vi "logic settings buffer.vi"(0 "output settings":T5, 1 "Rules":T6=[{"state rules"=[{"next state"=0, "conditions"=[], "number of conditions"=1, "Rule name"="New rule"}], "State name"="New state"}] {"state rules"."number of conditions" min=1 step=1; "state rules"."conditions"."Data average interval" min=0.0 format="%^#_3g"; "state rules"."conditions"."sensors and variables" items=["Elapsed time in current state"]; "state rules"."next state" items=["down flow", "Backwash", ""]}, 3 "output descriptions":string[][](array[string]), 4 "index":i32, 5 "Plant  state":i16(ring), 6 "Elapsed time in current state":dbl format="%.2f", 7 "command":T11=enum."write all", 8 "Set Points":T2[](array[typedef])=[{"name"="", "unit"="", "value"=0.0, "Type"=enum."Constant", "variable"={"selected sensors"=[], "selected set points"=[], "VI"=path "", "Data average interval"=0.0, "code ref"=refnum}}] {"value" format="%#_6p"; "variable"."Data average interval" min=0.0 format="%^#_3g"}, 11 "rule file in":path) -> (10 "Setpoint match":T1[](array[typedef]), 12 "Set Points out":T2[](array[typedef])=[{"name"="", "unit"="", "value"=0.0, "Type"=enum."Constant", "variable"={"selected sensors"=[], "selected set points"=[], "VI"=path "", "Data average interval"=0.0, "code ref"=refnum}}] {"value" format="%#_6p"; "variable"."Data average interval" min=0.0 format="%^#_3g"}, 13 "rule file out":path, 14 "ouput settings out":T5, 15 "Rules out":T6=[{"state rules"=[{"next state"=0, "conditions"=[], "number of conditions"=1, "Rule name"="New rule"}], "State name"="New state"}] {"state rules"."number of conditions" min=1 step=1; "state rules"."conditions"."Data average interval" min=0.0 format="%^#_3g"; "state rules"."conditions"."sensors and variables" items=["Elapsed time in current state"]; "state rules"."next state" items=["down flow", "Backwash", ""]}, 17 "output descriptions out":string[][](array[string]), 18 "code error array":errorcluster[](array[cluster]), 19 "Plant  state out":u16(ring)=1)   [LabVIEW 2012]
uses:
  logic buffer cmd.ctl
  rules.ctl
  State rules.ctl
  rule.ctl
  condition.ctl
  greater or less.ctl
  Output control.ctl
  variable setpoint.ctl
  data ave interval.ctl
  type specifier for control code.ctl
  setpoint match.ctl
  DAQ configuration/Sensor buffer command.ctl
  file/file action.ctl
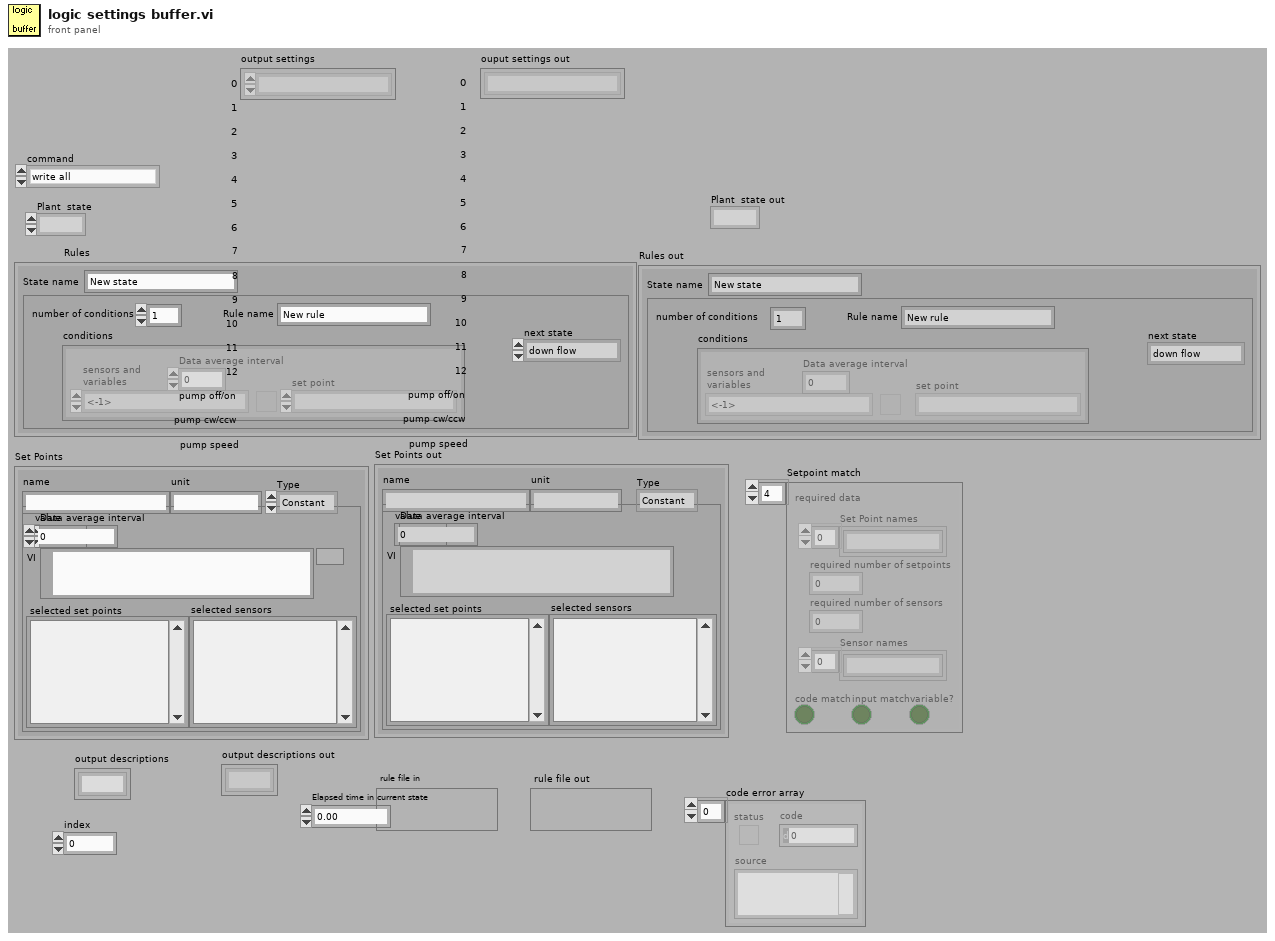
[diagram p1: front panel]
types:
  T1 = typedef "setpoint match.ctl" = cluster{"required data":cluster{"Set Point names":string[], "required number of setpoints":u8, "required number of sensors":u8, "Sensor names":string[]}, "input match":bool, "code match":bool, "variable?":bool}
  T2 = typedef "variable setpoint.ctl" = cluster{"name":string, "unit":string, "value":dbl, "Type":enum16{"Constant", "Variable"}, "variable":cluster{"selected sensors":i32[], "selected set points":i32[], "VI":path, "Data average interval":T3, "code ref":T4}}
  T3 = typedef "data ave interval.ctl" = dbl
  T4 = typedef "type specifier for control code.ctl" = refnum<vi>
  T5 = typedef "Output control.ctl" = u16[][]
  T6 = typedef "rules.ctl" = T7[]
  T7 = typedef "State rules.ctl" = cluster{"state rules":T8[], "State name":string}
  T8 = typedef "rule.ctl" = cluster{"next state":u16, "conditions":T9[], "number of conditions":u8, "Rule name":string}
  T9 = typedef "condition.ctl" = cluster{"> or <":T10, "set point":i32, "sensors and variables":i32, "Data average interval":dbl}
  T10 = typedef "greater or less.ctl" = bool
  T11 = typedef "logic buffer cmd.ctl" = enum16{"read", "write ouput settings", "write rules", "write setpoints", "write output descriptions", "write all", "calculate setpoints", "save", "open", "Load all setpoint code", "Load one setpoint code", "Configure one setpoint code"}
  T12 = typedef "Sensor buffer command.ctl" = enum16{"read average", "read recent", "read all", "write", "configure", "clear"}
  T13 = typedef "file action.ctl" = enum16{"Save", "Open"}
  T14 = typedef "Sensor data.ctl" = cluster{" Sensor array":T15[], "Time":dbl}
  T15 = typedef "sensor cluster.ctl" = cluster{"voltage":sgl, "scaled":sgl, "units":string, "Out of Range":bool}
  T16 = cluster{"Set Points out":T2[], "Rules":T6, "s? t:f":T5, "output descriptions":string[][]}
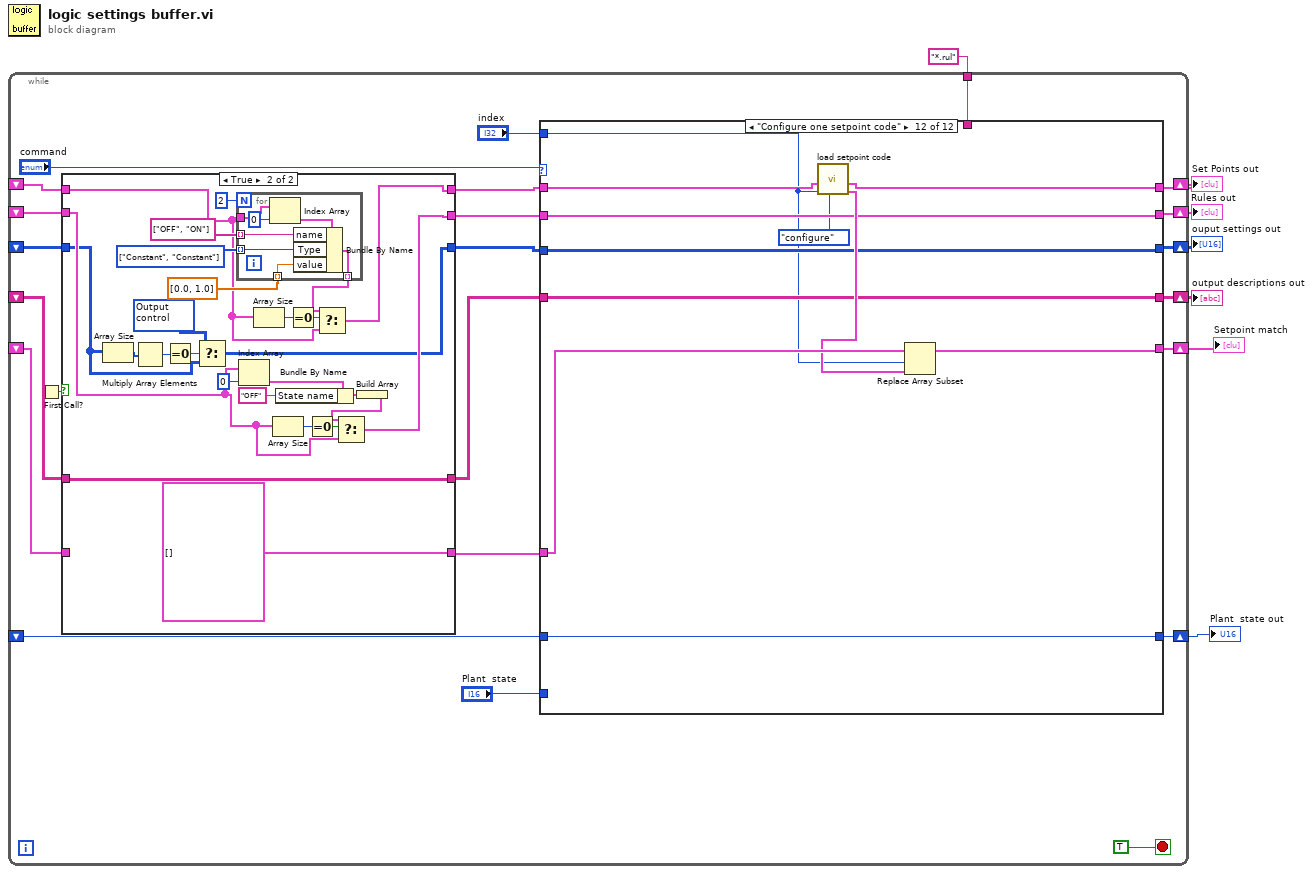
[diagram p0: block diagram]
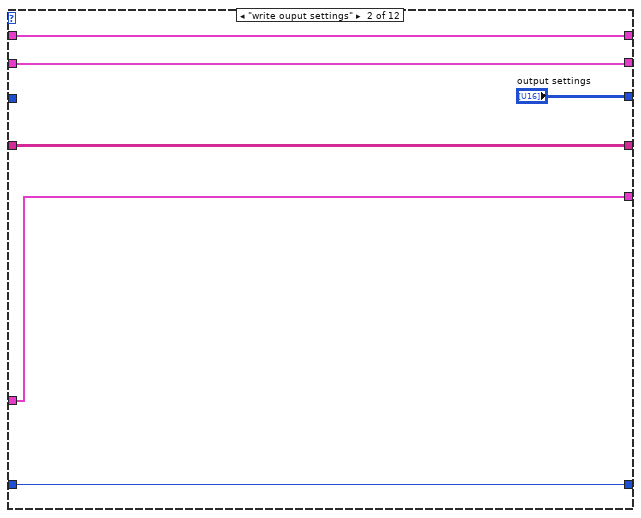
[diagram p4: hidden frame]
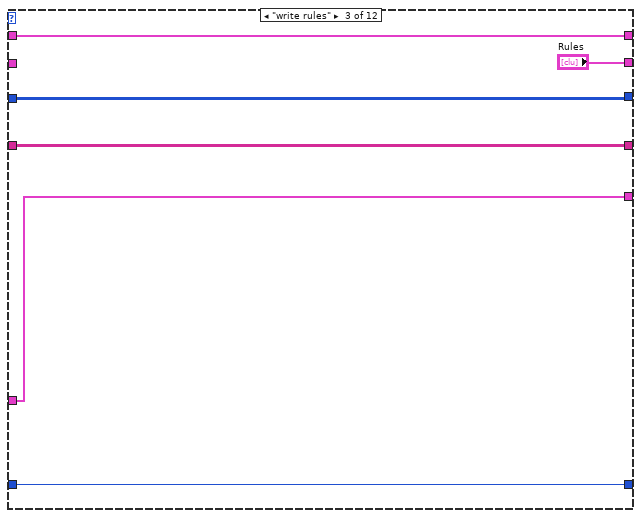
[diagram p5: hidden frame]
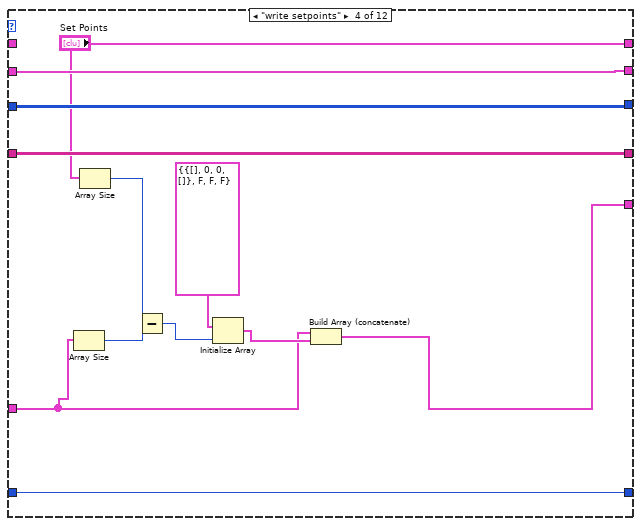
[diagram p6: hidden frame]
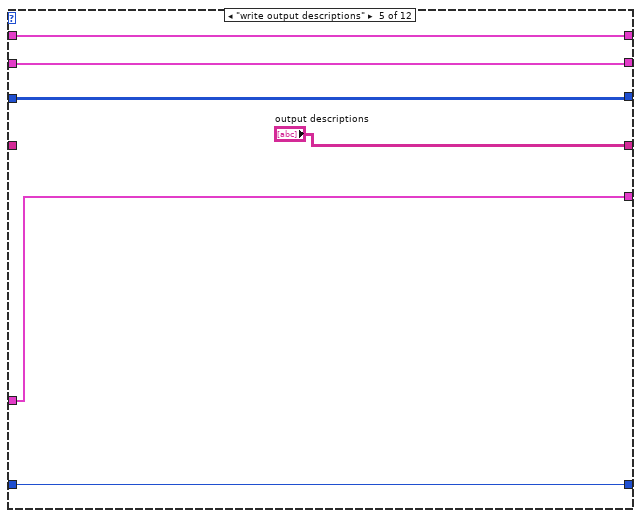
[diagram p7: hidden frame]
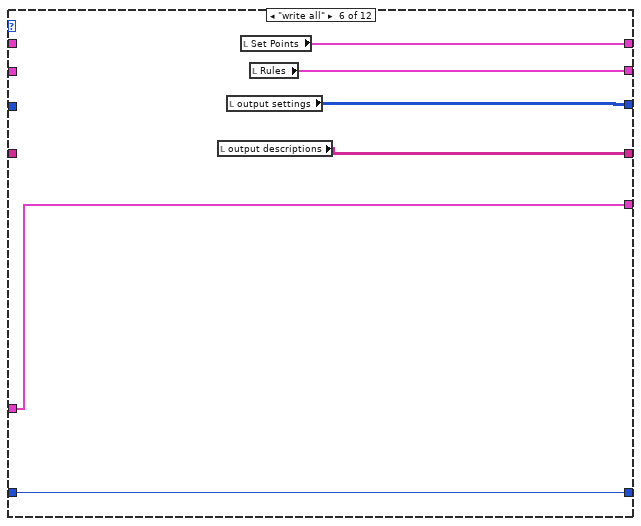
[diagram p8: hidden frame]
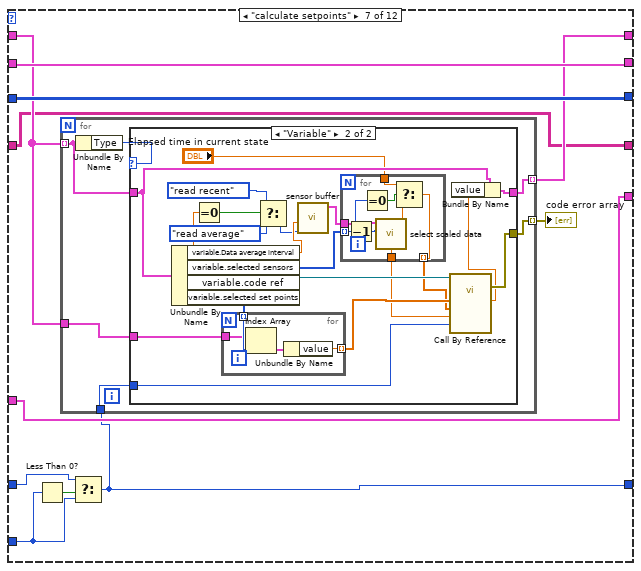
[diagram p9: hidden frame]
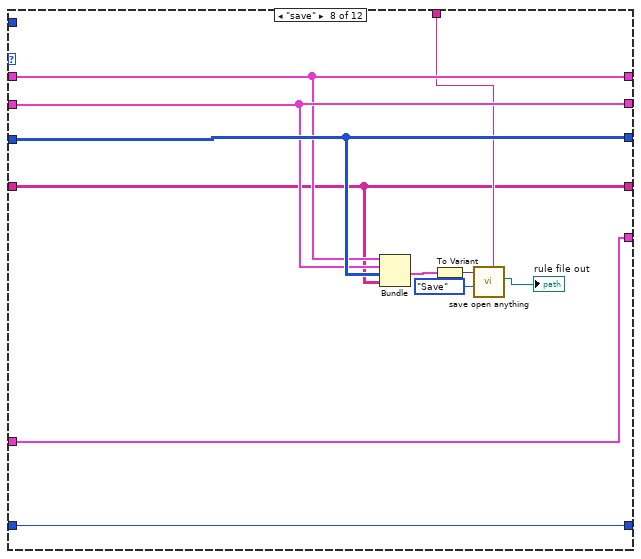
[diagram p11: hidden frame]
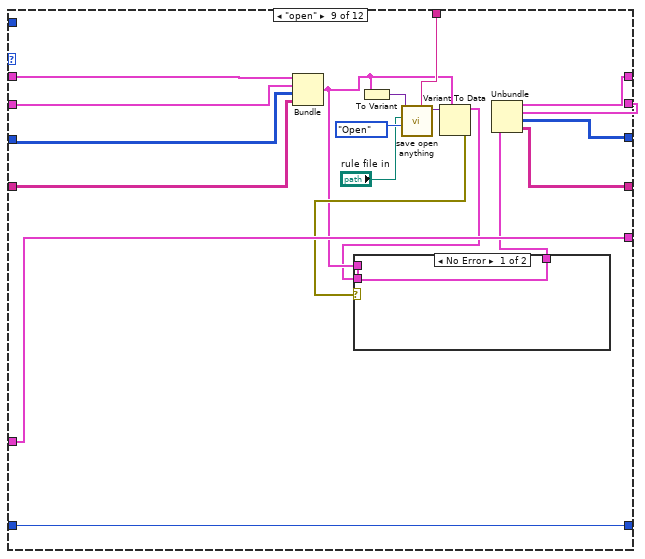
[diagram p12: hidden frame]
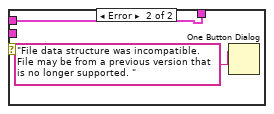
[diagram p13: hidden frame]
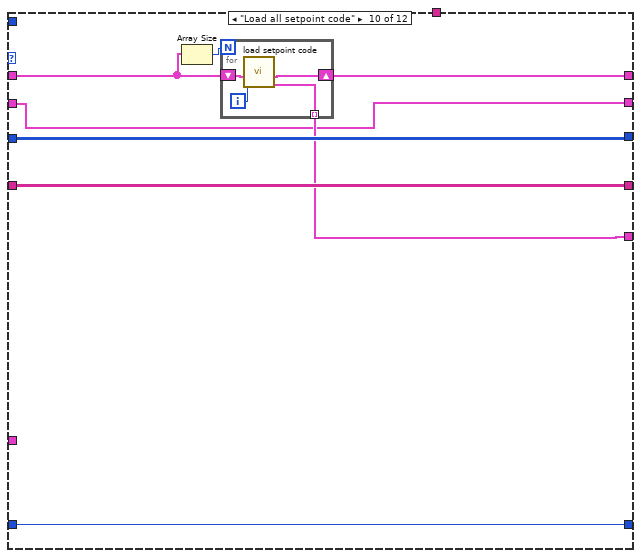
[diagram p14: hidden frame]
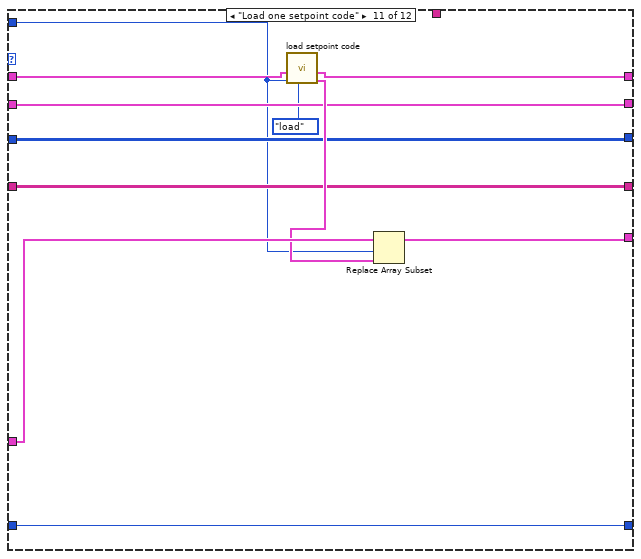
[diagram p15: hidden frame]
diagram:
  n1 = while {
    shift-right: [w29] -> w6
    shift-left: _ -> [w21]
    shift-right: [w30] -> w7
    shift-left: _ -> [w23]
    shift-right: [w15] -> w5
    shift-left: _ -> [w19]
    tunnel: "*.rul" ("pattern") -> [w27]
    shift-right: [w18] -> w3
    shift-left: _ -> [w17]
    shift-right: [w14] -> w2
    shift-left: _ -> [w12]
    shift-right: [w10] -> w1
    shift-left: _ -> [w11]
    stop <- TRUE stop-if-true
    n2 = First Call?() -> (First Call?: T/F=w25:bool)
    n3 = case shown="True" w25 {
      tunnel: [w35 w39] -> w24
      tunnel: w23 -> [w35 w38]
      tunnel: [w34 w40] -> w22
      tunnel: w21 -> [w34 w41]
      tunnel: [w33 w42] -> w20
      tunnel: w19 -> [w33 w43]
      tunnel: [w32 w37] -> w16
      tunnel: w17 -> [w32 w37]
      tunnel: [w31 T1[] [] ("Setpoint match")] -> w13
      tunnel: w12 -> [w31 _]
      frame False {
      }
      frame True {
        w52 = enum16{"Constant", "Variable"}[] [enum."Constant", enum."Constant"] items=["Constant", "Variable"]
        w58 = T5 [[0], [0], [0], [0], [0], [0], [0], [0], [0], [0], [0], [0], [0], [0], [0], [0], [0], [0], [0], [0], [0], [0], [0], [0], [0], [0], [0], [0], [0], [0], [0], [0]] items=[""] ("s? t:f")
        n4 = Array Size(array=w38) -> (size(s)=w61:i32[])
        n5 = Multiply Array Elements(1:w61) -> (0:w60:i32)
        n6 = Equal To 0?(x=w60) -> (x = 0?=w59:bool)
        n7 = Select(t=w58, s=w59, f=w38) -> (s? t:f=w39:T5)
        n8 = for {
          N: 2 -> [_]
          tunnel: w43 -> [w64]
          tunnel: [w68] -> w54 mode=indexing
          tunnel: string[] ["OFF", "ON"] -> [w67] mode=indexing
          tunnel: w52 -> [w66] mode=indexing
          tunnel: dbl[] [0.0, 1.0] -> [w65] mode=indexing
          n9 = Index Array(array=w64, index=0) -> (element=w62:T2)
          n10 = Bundle By Name(cluster=w62, "name"=w67, "Type"=w66, "value"=w65) -> (w68:T2)
        }
        n11 = Index Array(array=w41, index=0) -> (element=w47:T7)
        n12 = Array Size(array=w43) -> (size(s)=w56:i32)
        n13 = Array Size(array=w41) -> (size(s)=w50:i32)
        n14 = Bundle By Name(cluster=w47, "State name"="OFF") -> (w46:T7)
        n15 = Equal To 0?(x=w56) -> (x = 0?=w57:bool)
        n16 = Equal To 0?(x=w50) -> (x = 0?=w49:bool)
        n17 = Select(t=w54, s=w57, f=w43) -> (s? t:f=w42:T2[])
        n18 = Build Array(w46) -> (w45:T7[])
        n19 = Select(t=w45, s=w49, f=w41) -> (s? t:f=w40:T6)
      }
    }
    n20 = case shown="\"Configure one setpoint code\"" "command" {
      tunnel: [w73 "output settings" w85 w97 w102 w108 w121 w168 w180 w197 w209 w220] -> w30
      tunnel: [w74 w80 "Rules" w98 w103 w109 w120 w167 w184 w194 w210 w221] -> w29
      tunnel: w22 -> [w74 w80 _ w98 w103 _ w120 w167 w187 w194 w210 w221]
      tunnel: w24 -> [w73 _ w85 w97 w102 _ w121 w168 w186 w197 w209 w220]
      tunnel: [w72 w79 w84 "Set Points" w104 w110 w119 w166 w179 w198 w214 w225] -> w15
      tunnel: w20 -> [w72 w79 w84 _ w104 _ w118 w166 w185 w199 w215 w226]
      tunnel: w27 -> [_ _ _ _ _ _ _ w165 w182 _ _ _]
      tunnel: [w71 w77 w83 w96 "output descriptions" w107 w116 w162 w177 w196 w208 w219] -> w18
      tunnel: w16 -> [w71 w77 w83 w96 _ _ w116 w162 w178 w196 w208 w219]
      tunnel: [w70 w76 w82 w88 w100 w106 w115 w161 w176 w195 w212 w223] -> w14
      tunnel: w13 -> [w70 w76 w82 w89 w100 w106 w115 w161 w176 _ w213 w224]
      tunnel: w11 -> [w69 w75 w81 w87 w99 w105 w112 w160 w171 w193 w207 w218]
      tunnel: [w69 w75 w81 w87 w99 w105 w113 w160 w171 w193 w207 w218] -> w10
      tunnel: "Plant  state" -> [_ _ _ _ _ _ w111 _ _ _ _ _]
      tunnel: "index" -> [_ _ _ _ _ _ _ _ _ _ w205 w216]
      frame "read", Default {
      }
      frame "write ouput settings" {
      }
      frame "write rules" {
      }
      frame "write setpoints" {
        n21 = Array Size(array=w89) -> (size(s)=w92:i32)
        n22 = Array Size(array="Set Points") -> (size(s)=w94:i32)
        n23 = Subtract(x=w94, y=w92) -> (x-y=w93:i32)
        n24 = Initialize Array(T1 {"required data"={"Set Point names"=[], "required number of setpoints"=0, "required number of sensors"=0, "Sensor names"=[]}, "input match"=FALSE, "code match"=FALSE, "variable?"=FALSE} ("setpoint match"), w93) -> (w90:T1[])
        n25 = Build Array (concatenate)(w89, w90) -> (w88:T1[])
      }
      frame "write output descriptions" {
      }
      frame "write all" {
        n26 = local read "output descriptions"() -> (w107:string[][])
        n27 = local read "output settings"() -> (w108:T5)
        n28 = local read "Set Points"() -> (w110:T2[])
        n29 = local read "Rules"() -> (w109:T6)
      }
      frame "calculate setpoints" {
        n30 = Less Than 0?(x=w111) -> (x < 0?=w114:bool)
        n31 = Select(t=w112, s=w114, f=w111) -> (s? t:f=w113:i16)
        n32 = for {
          tunnel: [w127] -> w117 mode=indexing
          tunnel: w118 -> [w125] mode=indexing
          tunnel: [w124] -> w119 mode=indexing
          tunnel: w118 -> [w123]
          tunnel: w113 -> [w122]
          n33 = Unbundle By Name(w125) -> ("Type"=w126:enum16{"Constant", "Variable"})
          n34 = case shown="\"Variable\"" w126 {
            tunnel: [_ w147] -> w127
            tunnel: w122 -> [_ w146]
            tunnel: w125 -> [w128 w132]
            tunnel: [w128 w133] -> w124
            tunnel: w123 -> [_ w134]
            frame "Constant", Default {
            }
            frame "Variable" {
              n35 = Unbundle By Name(w132) -> ("variable.Data average interval"=w138:T3, "variable.selected sensors"=w142:i32[], "variable.code ref"=w145:T4, "variable.selected set points"=w144:i32[])
              n36 = Equal To 0?(x=w138) -> (x = 0?=w139:bool)
              n37 = for {
                tunnel: w144 -> [w159] mode=indexing
                tunnel: [w157] -> w141 mode=indexing
                tunnel: w134 -> [w156]
                n38 = Index Array(array=w156, index=w159) -> (element=w158:T2)
                n39 = Unbundle By Name(w158) -> ("value"=w157:dbl)
              }
              n40 = Select(t=Sensor_buffer_command."read recent" ("command"), s=w139, f=Sensor_buffer_command."read average" ("command")) -> (s? t:f=w137:T12)
              n41 = call "sensor buffer.vi"("command"=w137, "smooth interval (s)"=w138) -> ("Sensor Data smoothed"=w143:T14)  [unwired: 3 in, 2 out]
              n42 = for {
                tunnel: w143 -> [w155]
                tunnel: w142 -> [w149] mode=indexing
                tunnel: [w150] -> w130 mode=indexing
                tunnel: [w154] -> w140
                tunnel: "Elapsed time in current state" -> [w152]
                n43 = Decrement(x=w149) -> (x-1=w148:i32)
                n44 = Equal To 0?(x=w149) -> (x = 0?=w153:bool)
                n45 = call "select scaled data.vi"("Sensor index"=w148, "Sensor Data"=w155) -> ("scaled"=w151:sgl, "Time"=w154:dbl)  [unwired: 4 in, 4 out]
                n46 = Select(t=w152, s=w153, f=w151) -> (s? t:f=w150:dbl)
              }
              n47 = call-by-ref "?"(reference=w145, "State"=w146, "Time"=w140, "Sensor Values"=w130, "Set Points"=w141) -> (error out=w147:errorcluster, "fraction on"=w131:dbl)  [unwired: 3 in, 2 out]
              n48 = Bundle By Name(cluster=w132, "value"=w131) -> (w133:T2)
            }
          }
        }
        "code error array" <- w117
      }
      frame "save" {
        n49 = Bundle("Set Points out"=w166, "Rules"=w167, "s? t:f"=w168, "output descriptions"=w162) -> (w169:T16)  [unwired: 1 in]
        n50 = To Variant(anything=w169) -> (Variant=w170:variant)
        n51 = call "save open anything.vi"("Variant"=w170, "Action"=file_action."Save", "pattern"=w165) -> ("new file path"=→"rule file out":path)  [unwired: 4 in, 3 out]
      }
      frame "open" {
        n52 = Bundle("Set Points out"=w185, "Rules"=w187, "s? t:f"=w186, "output descriptions"=w178) -> (w174:T16)  [unwired: 1 in]
        n53 = To Variant(anything=w174) -> (Variant=w188:variant)
        n54 = call "save open anything.vi"("Variant"=w188, "file path"="rule file in", "Action"=file_action."Open", "pattern"=w182) -> ("Variant out"=w189:variant)  [unwired: 3 in, 3 out]
        n55 = Variant To Data(type=w174, Variant=w189) -> (data=w173:T16, error out=w175:errorcluster)  [unwired: 1 in]
        n56 = case shown="No Error" w175 {
          tunnel: [w190 w191] -> w172
          tunnel: w173 -> [_ _]
          tunnel: w174 -> [w190 w191]
          frame No Error {
          }
          frame Error {
            n57 = One Button Dialog(message="File data structure was incompatible. File may be from a previous version that is no longer supported. ") -> ()  [unwired: 1 in, 1 out]
          }
        }
        n58 = Unbundle(w172) -> ("Set Points out"=w179:T2[], "Rules"=w184:T6, "s? t:f"=w180:T5, "output descriptions"=w177:string[][])
      }
      frame "Load all setpoint code" {
        n59 = Array Size(array=w199) -> (size(s)=w200:i32)
        n60 = for {
          N: w200 -> [_]
          shift-right: [w202] -> w198
          shift-left: w199 -> [w203]
          tunnel: [w201] -> w195 mode=indexing
          i -> [w204]
          n61 = call "load setpoint code.vi"("index"=w204, "Set Points"=w203) -> ("setpoint match"=w201:T1, "Set Points out"=w202:T2[])  [unwired: 8 in]
        }
      }
      frame "Load one setpoint code" {
        n62 = call "load setpoint code.vi"("Load or config"=enum16{"load", "configure"}."load", "index"=w205, "Set Points"=w215) -> ("setpoint match"=w211:T1, "Set Points out"=w214:T2[])  [unwired: 7 in]
        n63 = Replace Array Subset(array=w213, new element=w211, index=w205) -> (w212:T1[])
      }
      frame "Configure one setpoint code" {
        n64 = call "load setpoint code.vi"("Load or config"=enum16{"load", "configure"}."configure", "index"=w216, "Set Points"=w226) -> ("setpoint match"=w222:T1, "Set Points out"=w225:T2[])  [unwired: 7 in]
        n65 = Replace Array Subset(array=w224, new element=w222, index=w216) -> (w223:T1[])
      }
    }
  }
  "Rules out" <- w6
  "ouput settings out" <- w7
  "Set Points out" <- w5
  "output descriptions out" <- w3
  "Setpoint match" <- w2
  "Plant  state out" <- w1
